vi "get_destination.vi"(8 "error in (no error)":errorcluster, 11 "HGF_Visitor":refnum<class "HGF_Visitor.lvclass">) -> (0 "error out":errorcluster, 2 "destination":refnum<class "HGF_TriggeredEvent.lvclass">, 3 "dup HGF_Visitor":refnum<class "HGF_Visitor.lvclass">)   [LabVIEW 2014, in "HGF_BaseClasses.lvlib" / "HGF_Visitor.lvclass"]
doc: "This VI returns a HGF_TriggeredEvent where the visitor would like to go after visiting the visitable."
uses:
  HGF_Visitor.lvclass
  HGF_TriggeredEvent/HGF_TriggeredEvent.lvclass
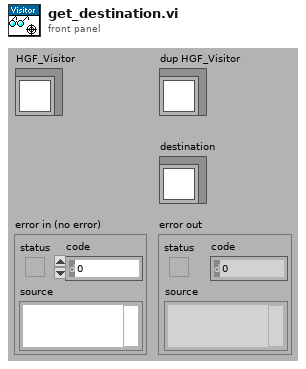
[diagram p1: front panel]
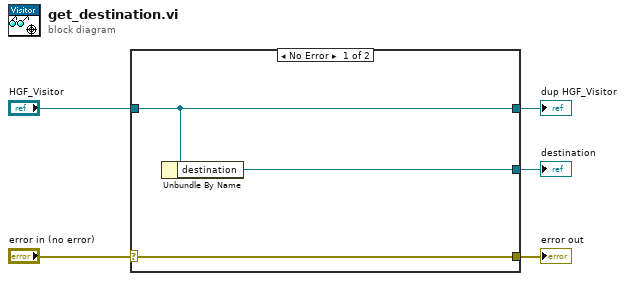
[diagram p0: block diagram]
diagram:
  n1 = case shown="No Error" "error in (no error)" {
    selector: "error in (no error)" -> [w8 w9]
    tunnel: [w8 w9] -> w4
    tunnel: [w7 w10] -> w2
    tunnel: "HGF_Visitor" -> [w7 w10]
    tunnel: [w6 _] -> w1
    frame No Error {
      n2 = Unbundle By Name(w7) -> ("destination"=w6:refnum<class "HGF_TriggeredEvent.lvclass">)
    }
    frame Error {
    }
  }
  "error out" <- w4
  "dup HGF_Visitor" <- w2
  "destination" <- w1
